vi "AI RAG Close.vi"(8 "error in":errorcluster) -> (0 "error out":errorcluster)   [LabVIEW 2023, in "LabVIEW RAG.lvlib"]
uses:
  LabVIEW RAG.lvlib
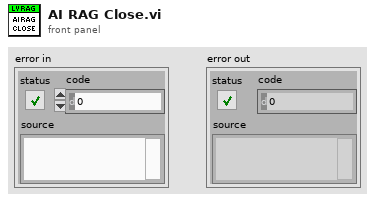
[diagram p1: front panel]
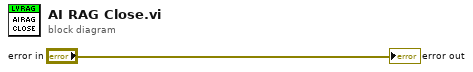
[diagram p0: block diagram]
diagram:
  "error out" <- "error in"
